vi "Write Address.vi"(8 "error in":errorcluster, 10 "Address":string[](array[string]), 11 "CN79000 in":refnum<class "CN79000.lvclass">) -> (0 "error out":errorcluster, 3 "CN79000 out":refnum<class "CN79000.lvclass">)   [LabVIEW 2012, in "CN79000.lvclass"]
uses:
  CN79000.lvclass
  CN79000.lvclass/CN79000.ctl
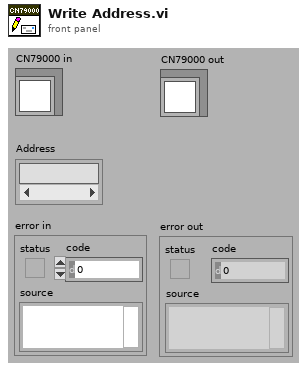
[diagram p1: front panel]
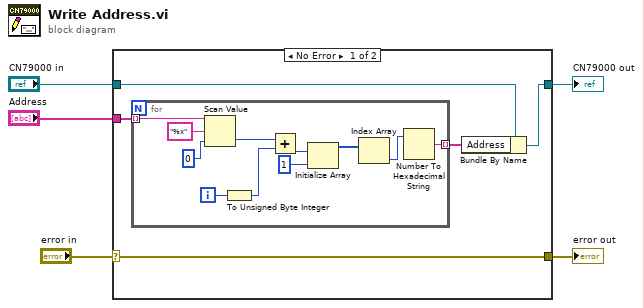
[diagram p0: block diagram]
diagram:
  n1 = case shown="No Error" "error in" {
    selector: "error in" -> [w10 w22]
    tunnel: [w10 w22] -> w4
    tunnel: [w8 w23] -> w2
    tunnel: "CN79000 in" -> [w9 w23]
    tunnel: "Address" -> [w6 _]
    frame No Error {
      n2 = for {
        tunnel: [w13] -> w7 mode=indexing
        tunnel: w6 -> [w12] mode=indexing
        i -> [w11]
        n3 = Scan Value(string=w12, format string="%x", default (0 dbl)=u8 0) -> (value=w18:u8)  [unwired: 1 out]
        n4 = To Unsigned Byte Integer(number=w11) -> (unsigned 8bit integer=w21:u8)
        n5 = Add(x=w18, y=w21) -> (x+y=w19:u8)
        n6 = Initialize Array(w19, 1 ("dimension size")) -> (w15:u8[])
        n7 = Index Array(array=w15) -> (element=w14:u8)  [unwired: 1 in]
        n8 = Number To Hexadecimal String(2:w14) -> (0:w13:string)  [unwired: 1 in]
      }
      n9 = Bundle By Name(cluster=w9, "Address"=w7) -> (w8:refnum<class "CN79000.lvclass">)
    }
    frame Error {
    }
  }
  "error out" <- w4
  "CN79000 out" <- w2
